vi "WPI_CameraSet Image Compression.vi"(8 "error in (no error)":errorcluster, 10 "Compression":i32 min=0 max=100, 11 "CameraDevRef":T1={"Camera Address"="192.168.0.90", "CameraStatus"={"status"=FALSE, "code"=0, "source"=""}}) -> (0 "error out":errorcluster, 3 "CameraDevRef Out":T1)   [LabVIEW 2017]
doc: "Sets the level of compression of the image from the camera. The higher the level of image compression, the smaller the file size but the lower the image quality.\n\nThis software is licensed. Open the labview\\readme\\WPI Robotics Library Open Source License.txt file for more information."
uses:
  <vilib>/Rock Robotics/WPI/Camera/WPI_CameraDevRef.ctl
  <vilib>/Rock Robotics/WPI/Camera/WPI_CameraSettings Operations.ctl
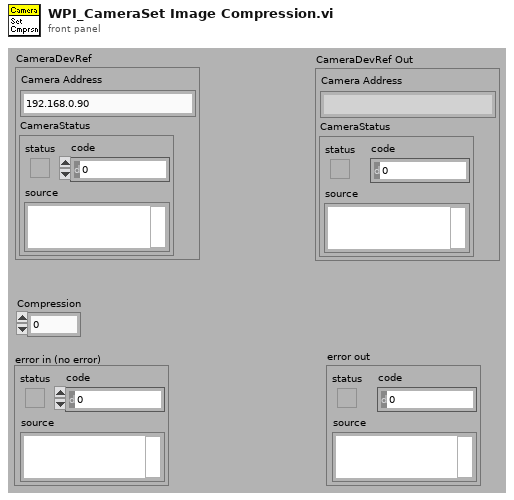
[diagram p1: front panel]
types:
  T1 = typedef "WPI_CameraDevRef.ctl" = cluster{"Camera Address":string, "CameraStatus":errorcluster}
  T2 = typedef "WPI_CameraSettings Operations.ctl" = enum16{"Udate FPS", "Update Compression", "Update Size", "Update White Balance", "Update Brightness", "Update Sharpness", "Update Exposure", "Update Exposure Value", "Update Color Level", "Update Exp Priority", "Update Color Enable", "Update JPG", "Update MJPG", "Read and Clear", "Read", "Init"}
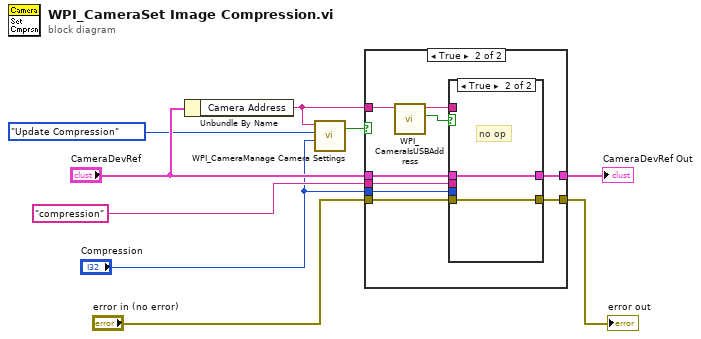
[diagram p0: block diagram]
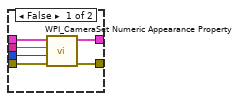
[diagram p3: hidden frame]
diagram:
  n1 = Unbundle By Name("CameraDevRef") -> ("Camera Address"=w1:string)
  n2 = call <vilib>:"WPI_CameraManage Camera Settings.vi"("Value"="Compression", "Operation"=WPI_CameraSettings_Operations."Update Compression", "Camera IP"=w1) -> ("Changed"=w5:bool)  [unwired: 7 in, 1 out]
  n3 = case shown="True" w5 {
    tunnel: "CameraDevRef" -> [w10 w20]
    tunnel: "compression" ("Property Name") -> [_ w19]
    tunnel: "Compression" -> [_ w18]
    tunnel: [w10 w17] -> w8
    tunnel: "error in (no error)" -> [w11 w16]
    tunnel: [w11 w15] -> w6
    tunnel: w1 -> [_ w14]
    frame False {
    }
    frame True {
      n4 = call <vilib>:"WPI_CameraIsUSBAddress.vi"("Camera Address In"=w14) -> ("USB?"=w13:bool, "Camera Address Out"=w12:string)  [unwired: 8 in, 1 out]
      n5 = case shown="True" w13 {
        tunnel: w20 -> [w26 w28]
        tunnel: w19 -> [w25 _]
        tunnel: w18 -> [w24 _]
        tunnel: [w23 w28] -> w17
        tunnel: w16 -> [w22 w27]
        tunnel: [w21 w27] -> w15
        tunnel: w12 -> [_ _]
        frame False {
          n6 = call <vilib>:"WPI_CameraSet Numeric Appearance Property.vi"("error in (no error)"=w22, "Value"=w24, "Property Name"=w25, "CameraDevRef"=w26) -> ("error out"=w21:errorcluster, "CameraDevRef out"=w23:T1)  [unwired: 6 out]
        }
        frame True {
          # "no op"
        }
      }
    }
  }
  "CameraDevRef Out" <- w8
  "error out" <- w6
